vi "UDP Named Service - Rotator Server.vi"() -> ()   [LabVIEW 2025]
doc: "Creates a named service and listens on the first available port. When a client connects to the service, it sends a response string to the client.\nAuthor: Scott Hannahs <sth@magnet.fsu.edu>\n\nThis software is licensed for use under the “MIT License\"\nCopyright (c) 2025 Scott Hannahs, sth@sth@magnet.sthnet.net\n\nPermission is hereby granted, free of charge, to any person obtaining a copy of this software and associated documentation files (the \"Software\"), to deal in the Software without restriction, including without limitation the rights to use, copy, modify, merge, publish, distribute, sublicense, and/or sell copies of the Software, and to permit persons to whom the Software is furnished to do so, subject to the following conditions: The above copyright notice and this permission notice shall be included in all copies or substantial portions of the Software.\n\nTHE SOFTWARE IS PROVIDED \"AS IS\", WITHOUT WARRANTY OF ANY KIND, EXPRESS OR IMPLIED, INCLUDING BUT NOT LIMITED TO THE WARRANTIES OF MERCHANTABILITY, FITNESS FOR A PARTICULAR PURPOSE AND NONINFRINGEMENT. IN NO EVENT SHALL THE AUTHORS OR COPYRIGHT HOLDERS BE LIABLE FOR ANY CLAIM, DAMAGES OR OTHER LIABILITY, WHETHER IN AN ACTION OF CONTRACT, TORT OR OTHERWISE, ARISING FROM, OUT OF OR IN CONNECTION WITH THE SOFTWARE OR THE USE OR OTHER DEALINGS IN THE SOFTWARE."
uses:
  <vilib>/Utility/error.llb/Trim Whitespace One-Sided.vi
panel:
  out "Port":u16
  out "String":string
  in  "Stop":bool
  # "Overview: Demonstrates the use of the UDP functions to initialize a named UDP service that can send data to a client VI.\nInstructions:\n1. Run the VI.\n2. Open UDP Named Service - Client.vi and follow the instructions on its front panel.\n3. Click Stop to stop the VI."
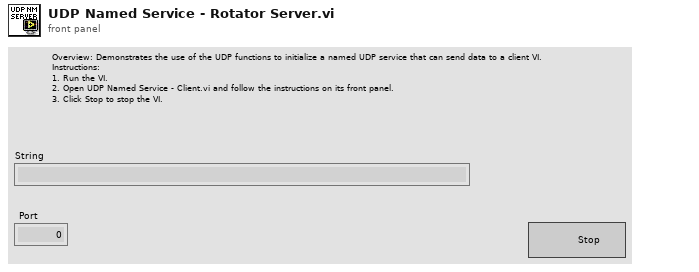
[diagram p1: front panel]
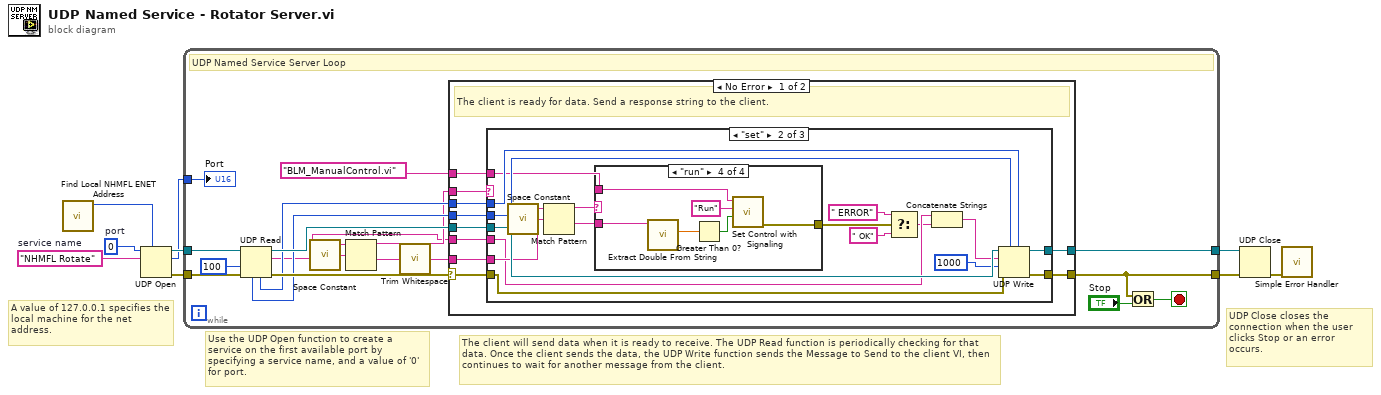
[diagram p0: block diagram]
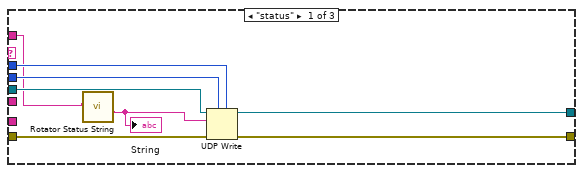
[diagram p2: hidden frame]
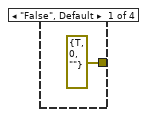
[diagram p3: hidden frame]
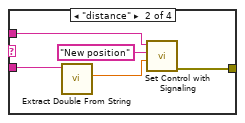
[diagram p4: hidden frame]
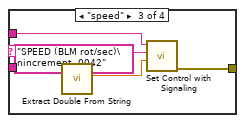
[diagram p5: hidden frame]
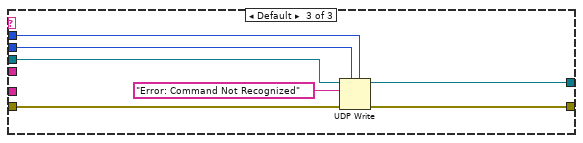
[diagram p6: hidden frame]
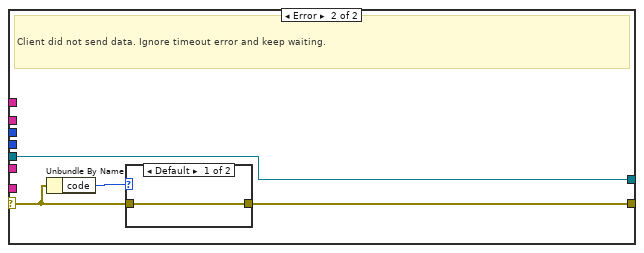
[diagram p7: hidden frame]
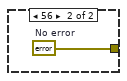
[diagram p8: hidden frame]
diagram:
  w2 = u16 0  # port
  w9 = "NHMFL Rotate"  # service name
  # "UDP Close closes the connection when the user clicks Stop or an error occurs."
  # "A value of 127.0.0.1 specifies the local machine for the net address."
  # "The client will send data when it is ready to receive. The UDP Read function is periodically checking for that data. Once the client sends the data, the UDP Write function sends the Message to Send to the client VI, then continues to wait for another message from the client."
  # "Use the UDP Open function to create a service on the first available port by specifying a service name, and a value of '0' for port."
  n1 = call "Find Local NHMFL ENET Address.vi"() -> ("Ethernet Address"=w1:u32)  [unwired: 9 in, 2 out]
  n2 = UDP Open(7:w1, 10:w9, 11:w2) -> (port=w8:refnum<k16>, 0:w7:errorcluster, 2:w4:u16)  [unwired: 2 in]
  n3 = while {
    tunnel: [w18] -> w5
    tunnel: w8 -> [w27]
    tunnel: w7 -> [w23]
    tunnel: [w24] -> w6
    tunnel: w4 -> [w21]
    stop <- w20 stop-if-true
    # "UDP Named Service Server Loop"
    n4 = UDP Read(connection ID=w27, timeout ms (25000)=100, 8:w23) -> (data out=w11:string, error out=w26:errorcluster, 3:w25:refnum<k16>, 4:w22:u16, 6:w16:u32)  [unwired: 1 in]
    n5 = call <vilib>:"Space Constant.vi"() -> ("String"=w12:string)
    n6 = Match Pattern(string=w11, regular expression=w12) -> (before substring=w15:string, after substring=w14:string)  [unwired: 1 in, 2 out]
    n7 = call <vilib>:"Trim Whitespace.vi"("string"=w14) -> ("trimmed string"=w13:string)  [unwired: 1 in]
    n8 = case shown="No Error" w26 {
      selector: w26 -> [w37 w90]
      tunnel: w25 -> [w34 w91]
      tunnel: [w36 w88] -> w18
      tunnel: [w35 w91] -> w24
      tunnel: w16 -> [w32 _]
      tunnel: w22 -> [w33 _]
      tunnel: w15 -> [w31 _]
      tunnel: w13 -> [w30 _]
      tunnel: w11 -> [w29 _]
      tunnel: "BLM_ManualControl.vi" -> [w28 _]
      frame No Error {
        # "The client is ready for data. Send a response string to the client."
        n9 = case shown="\"set\"" w31 {
          tunnel: w37 -> [w45 w63 w87]
          tunnel: [w44 w62 w86] -> w36
          tunnel: [w43 w61 w85] -> w35
          tunnel: w34 -> [w42 w60 w84]
          tunnel: w33 -> [w41 w59 w83]
          tunnel: w32 -> [w40 w58 w82]
          tunnel: w30 -> [_ w57 _]
          tunnel: w29 -> [_ w53 _]
          tunnel: w28 -> [w39 w46 _]
          frame "status" {
            n10 = call "Rotator Status String.vi"("VI Name"=w39) -> ("Status String"=w38:string)  [unwired: 9 in, 1 out]
            "String" <- w38
            n11 = UDP Write(address=w40, port or service name=w41, connection ID=w42, data in=w38, 8:w45) -> (error out=w44:errorcluster, 3:w43:refnum<k16>)  [unwired: 1 in]
          }
          frame "set" {
            n12 = call <vilib>:"Space Constant.vi"() -> ("String"=w56:string)
            n13 = Match Pattern(string=w57, regular expression=w56) -> (before substring=w55:string, after substring=w54:string)  [unwired: 1 in, 2 out]
            n14 = case shown="\"run\"" w55 {
              tunnel: w54 -> [_ w66 w71 w77]
              tunnel: w46 -> [_ w68 w73 w79]
              tunnel: [errorcluster {"status"=TRUE, "code"=0, "source"=""} ("error out") w65 w70 w76] -> w52
              frame "False", Default {
              }
              frame "distance" {
                n15 = call "Extract Double From String.vi"("string"=w66) -> ("floating pt. number"=w67:dbl)  [unwired: 3 in, 3 out]
                n16 = call "Set Control with Signaling.vi"("Value"=w67, "Control Name"="New position", "VI Name"=w68) -> ("error out"=w65:errorcluster)  [unwired: 8 in]
              }
              frame "speed" {
                n17 = call "Extract Double From String.vi"("string"=w71) -> ("floating pt. number"=w72:dbl)  [unwired: 3 in, 3 out]
                n18 = call "Set Control with Signaling.vi"("Value"=w72, "Control Name"="SPEED (BLM rot/sec)\nincrement .0042", "VI Name"=w73) -> ("error out"=w70:errorcluster)  [unwired: 8 in]
              }
              frame "run" {
                n19 = call "Extract Double From String.vi"("string"=w77) -> ("floating pt. number"=w78:dbl)  [unwired: 3 in, 3 out]
                n20 = Greater Than 0?(x=w78) -> (x > 0?=w75:bool)
                n21 = call "Set Control with Signaling.vi"("Value"=w75, "Control Name"="Run", "VI Name"=w79) -> ("error out"=w76:errorcluster)  [unwired: 8 in]
              }
            }
            n22 = Select(t=" ERROR", s=w52, f=" OK") -> (s? t:f=w48:string)
            n23 = Concatenate Strings(w53, w48) -> (w47:string)
            n24 = UDP Write(address=w58, port or service name=w59, connection ID=w60, data in=w47, 8:w63, 9:1000 ("timeout ms (25000)")) -> (error out=w62:errorcluster, 3:w61:refnum<k16>)
          }
          frame Default {
            n25 = UDP Write(address=w82, port or service name=w83, connection ID=w84, data in="Error: Command Not Recognized", 8:w87) -> (error out=w86:errorcluster, 3:w85:refnum<k16>)  [unwired: 1 in]
          }
        }
      }
      frame Error {
        # "Client did not send data. Ignore timeout error and keep waiting."
        n26 = Unbundle By Name(w90) -> ("code"=w89:i32)
        n27 = case shown="Default" w89 {
          tunnel: w90 -> [w92 _]
          tunnel: [w92 w93] -> w88
          frame Default {
          }
          frame 56 {
            w93 = errorcluster {"status"=FALSE, "code"=0, "source"=""}  # No error
          }
        }
      }
    }
    n28 = Or(x=w18, y="Stop") -> (x .or. y?=w20:bool)
    "Port" <- w21
  }
  n29 = UDP Close(connection ID=w6, 8:w5) -> (error out=w3:errorcluster)  [unwired: 1 out]
  n30 = call <vilib>:"Simple Error Handler.vi"("error in (no error)"=w3) -> ()  [unwired: 4 in, 5 out]
